vi "DataProcessingDraft.vi"() -> ()   [LabVIEW 2011]
doc: "Processes data from status data logs. Runs through it and finds each time we wrote to the log, and uses the number of times we wrote as the time (time stamps are acting funny). Then allows us to look at various pieces of data and zoom in and out as necessary.\n\n-By Elizabeth Mahon"
uses:
  2-Think/2 Typedefs/logger data.ctl
  2-Think/2 Typedefs/Which Boat.ctl
  2-Think/2 Typedefs/UTM Location.ctl
  2-Think/2 Typedefs/heading.ctl
  2-Think/2 Typedefs/rate of turn.ctl
  2-Think/2 Typedefs/robot velocity.ctl
  2-Think/2 Typedefs/pitch and roll.ctl
  2-Think/2 Typedefs/generalized sensor status.ctl
  2-Think/2 Typedefs/indicator LED.ctl
  2-Think/2 Typedefs/apparent wind direction.ctl
  2-Think/2 Typedefs/apparent wind speed.ctl
  2-Think/2 Typedefs/absolute wind direction.ctl
  2-Think/2 Typedefs/absolute wind speed.ctl
  0x2-OCU-Think Comm/0x2 Typedefs/Current Waypoint.ctl
  2-Think/2 Typedefs/UTM Circle.ctl
  2-Think/2 Typedefs/rudder angle.ctl
  2-Think/2 Typedefs/sail setpt.ctl
  0x2-OCU-Think Comm/0x2 Typedefs/manual override.ctl
  2-Think/2 Typedefs/setpoints to boat.ctl
panel:
  in  "Max time":dbl
  in  "Min time":dbl
  in  "Stop Viewing Data":bool
  in  "Choose graph to display":T1(tab)
  in  "Min Frequency":dbl
  in  "Max Frequency":dbl
  out "Code Speed":cluster{i32[], dbl[]}[](graph)
  out "Location":cluster{dbl[], dbl[]}(graph)
  out "Battery Voltage":cluster{i32[], dbl[]}(graph)
  in  "Min Velocity":dbl
  in  "Max Velocity":dbl
  out "Velocity":cluster{i32[], dbl[]}[](graph)
  in  "Min Angle":dbl
  in  "Max Angle":dbl
  out "Headings":cluster{i32[], dbl[]}[](graph)
  out "Rudder":cluster{i32[], dbl[]}(graph)
  out "Sail":cluster{i32[], dbl[]}(graph)
  in  "Data Log":T2 {"Current Waypoint Coords"."North" format="%#_10f"; "Current Waypoint Coords"."East" format="%#_8f"; "Robot Pitch/Roll"."Roll" format="%05.1f"; "Robot Pitch/Roll"."Pitch" format="%05.1f"; "Robot\nRate of Turn" format="%05.1f"; "Robot\nHeading" format="%05.1f"; "Robot UTM Location"."North" format="%#_10f"; "Robot UTM Location"."East" format="%#_8f"}
  # "Act and network frequency are always 0.\nAs far as I can tell, network frequency is never set, so of course it's 0.\nAct, while set, is in a sequence structure where the first frame has a while loop that only ends if we e-stop, so it'll never get set."
  # "Where Am I?"
  # "Path Planning"
  # "From Planning Functions"
  # "(this is not a cluster because subitems\nare generated in parallel code)"
  # "How Am I?"
  # "What's Around Me?"
  # "As Measured"
  # "As Measured"
  # "Loop Rates"
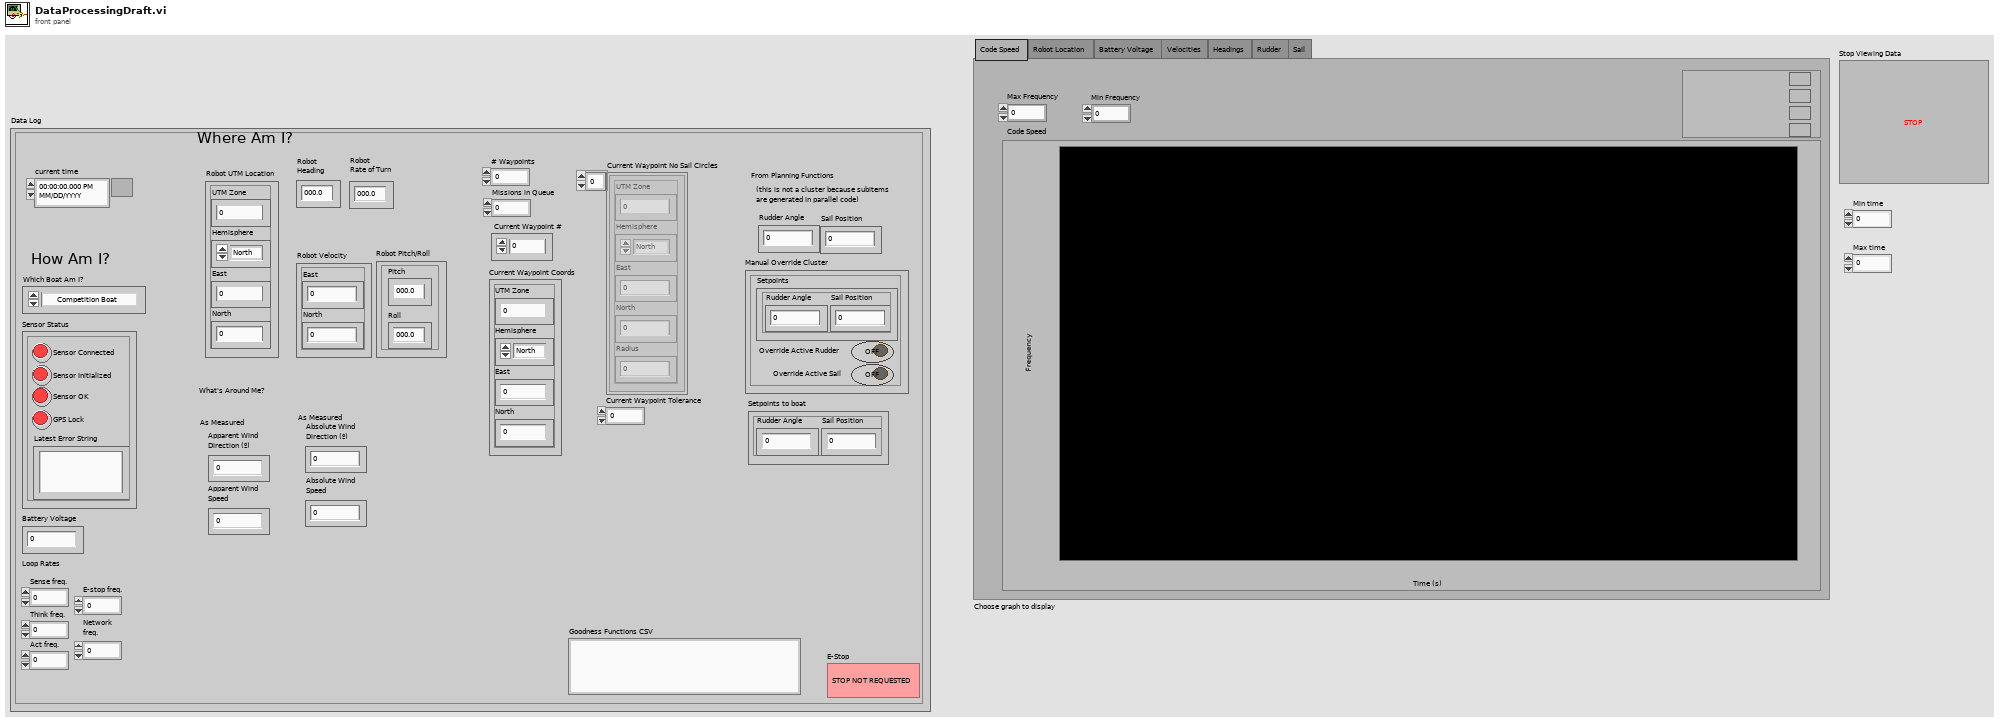
[diagram p1: front panel]
types:
  T1 = enum32{"Code Speed", "Robot Location", "Battery Voltage", "Velocities", "Headings", "Rudder", "Sail"}
  T2 = typedef "logger data.ctl" = cluster{"current time":timestamp, "Which Boat Am I?":T3, "Robot UTM Location":T4, "Robot\nHeading ":T5, "Robot\nRate of Turn":T6, "Robot Velocity":T7, "Robot Pitch/Roll":T8, "Sensor Status":T9, "Battery Voltage":dbl, "Sense freq.":dbl, "Think freq.":dbl, "Act freq.":dbl, "E-stop freq.":dbl, "Network \nfreq.":dbl, "Apparent Wind\nDirection (º)":T11, "Apparent Wind\nSpeed":T12, "Absolute Wind\nDirection (º)":T13, "Absolute Wind\nSpeed":T14, "Missions in Queue":i32, "# Waypoints":i32, " Current Waypoint #":T15, "Current Waypoint Coords":T4, "Current Waypoint Tolerance":dbl, "Current Waypoint No Sail Circles":T16[], "Rudder Angle":T17, "Sail Position":T18, "Manual Override Cluster":T19, "Setpoints to boat":T20, "E-Stop":bool, "Goodness Functions CSV":string}
  T3 = typedef "Which Boat.ctl" = enum16{"Competition Boat", "Small RC", "Simulation"}
  T4 = typedef "UTM Location.ctl" = cluster{"UTM Zone":dbl, "Hemisphere":enum16{"North", "South"}, "East":dbl, "North":dbl}
  T5 = typedef "heading.ctl" = dbl
  T6 = typedef "rate of turn.ctl" = dbl
  T7 = typedef "robot velocity.ctl" = cluster{"East":dbl, "North":dbl}
  T8 = typedef "pitch and roll.ctl" = cluster{"Pitch":dbl, "Roll":dbl}
  T9 = typedef "generalized sensor status.ctl" = cluster{"Sensor Connected":T10, "Sensor Initialized":T10, "Sensor OK":T10, "Latest Error String":string, "GPS Lock":T10}
  T10 = typedef "indicator LED.ctl" = bool
  T11 = typedef "apparent wind direction.ctl" = dbl
  T12 = typedef "apparent wind speed.ctl" = dbl
  T13 = typedef "absolute wind direction.ctl" = dbl
  T14 = typedef "absolute wind speed.ctl" = dbl
  T15 = typedef "Current Waypoint.ctl" = i32
  T16 = typedef "UTM Circle.ctl" = cluster{"UTM Zone":dbl, "Hemisphere":enum16{"North", "South"}, "East":dbl, "North":dbl, "Radius":dbl}
  T17 = typedef "rudder angle.ctl" = dbl
  T18 = typedef "sail setpt.ctl" = dbl
  T19 = typedef "manual override.ctl" = cluster{"Override Active Rudder":bool, "Setpoints":T20, "Override Active Sail":bool}
  T20 = typedef "setpoints to boat.ctl" = cluster{"Sail Position":T18, "Rudder Angle":T17}
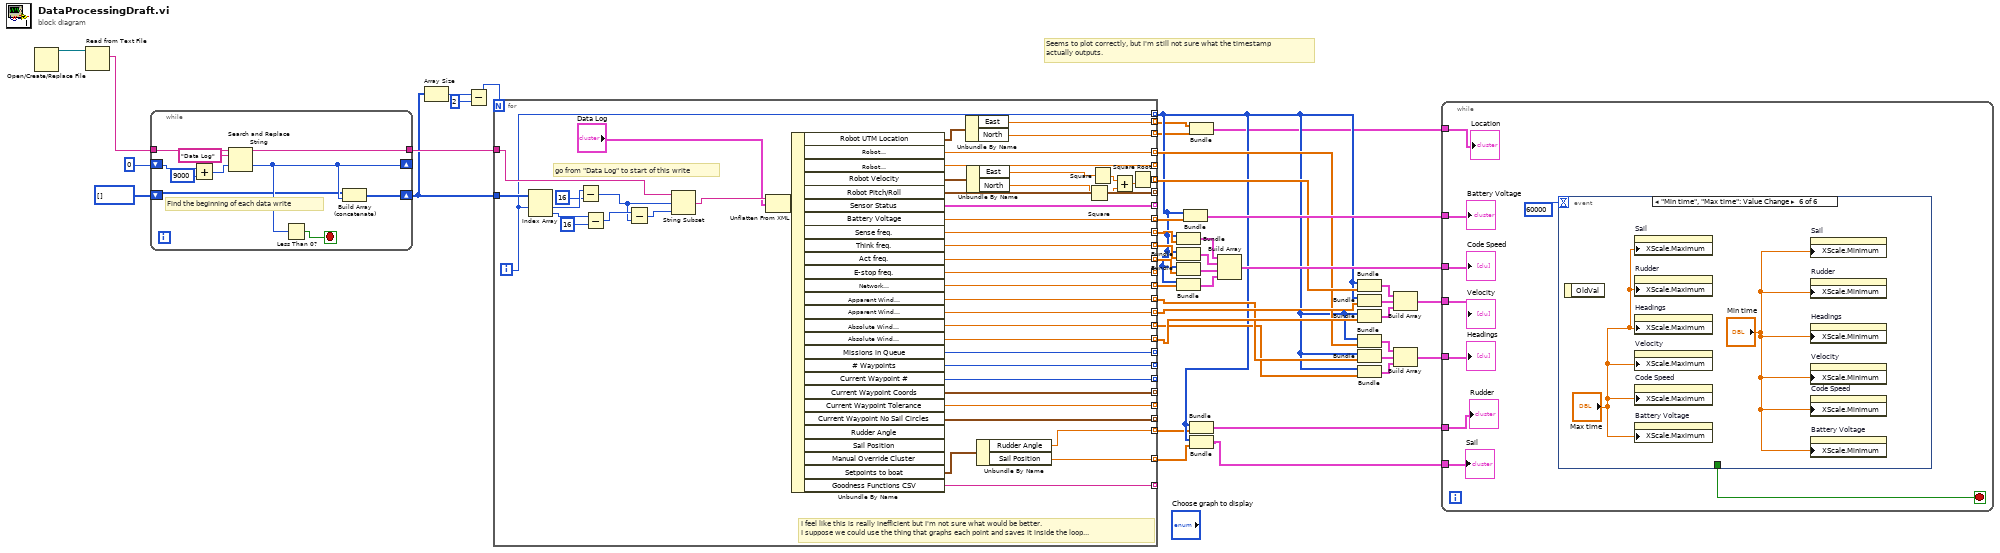
[diagram p0: block diagram]
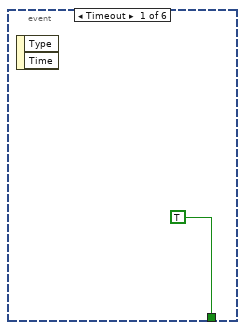
[diagram p2: hidden frame]
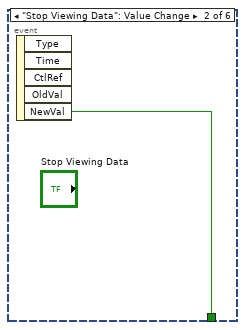
[diagram p3: hidden frame]
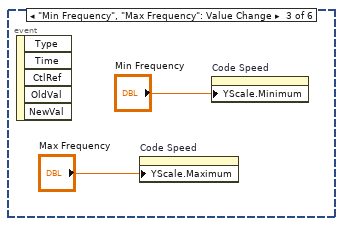
[diagram p4: hidden frame]
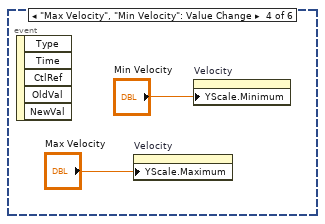
[diagram p5: hidden frame]
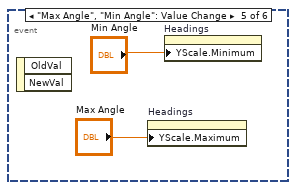
[diagram p6: hidden frame]
diagram:
  # "Seems to plot correctly, but I'm still not sure what the timestamp\nactually outputs."
  n1 = Open/Create/Replace File() -> (refnum out=w42:refnum<file>)  [unwired: 6 in, 2 out]
  n2 = Read from Text File(file (use dialog)=w42) -> (text=w41:string)  [unwired: 3 in, 3 out]
  n3 = while {
    tunnel: w41 -> [w51]
    shift-right: [w46] -> _
    shift-left: 0 ("offset past replacement") -> [w50]
    shift-right: [w45] -> w37
    shift-left: i32[] [] -> [w44]
    tunnel: [w43] -> w38
    stop <- w47 stop-if-true
    # "Find the beginning of each data write"
    n4 = Add(x=w50, y=9000) -> (x+y=w48:i32)
    n5 = Search and Replace String(input string=w51, search string="Data Log", offset=w48) -> (result string=w43:string, offset past replacement=w46:i32)  [unwired: 5 in, 2 out]
    n6 = Less Than 0?(x=w46) -> (x < 0?=w47:bool)
    n7 = Build Array (concatenate)(w44, w46) -> (w45:i32[])
  }
  n8 = Array Size(array=w37) -> (size(s)=w36:i32)
  n9 = Subtract(x=w36, y=2) -> (x-y=w35:i32)
  n10 = for {
    N: w35 -> [_]
    tunnel: w37 -> [w91]
    tunnel: w38 -> [w94]
    tunnel: [w87] -> w12 mode=indexing
    tunnel: [w86] -> _ mode=indexing
    tunnel: [w85] -> _ mode=indexing
    tunnel: [w84] -> _ mode=indexing
    tunnel: [w83] -> w23 mode=indexing
    tunnel: [w82] -> w21 mode=indexing
    tunnel: [w81] -> w20 mode=indexing
    tunnel: [w80] -> w19 mode=indexing
    tunnel: [w79] -> _ mode=indexing
    tunnel: [w78] -> w18 mode=indexing
    tunnel: [w77] -> w11 mode=indexing
    tunnel: [w76] -> w15 mode=indexing
    tunnel: [w75] -> w10 mode=indexing
    tunnel: [w74] -> w14 mode=indexing
    tunnel: [w73] -> _ mode=indexing
    tunnel: [w72] -> _ mode=indexing
    tunnel: [w71] -> _ mode=indexing
    tunnel: [w70] -> _ mode=indexing
    tunnel: [w69] -> _ mode=indexing
    tunnel: [w68] -> _ mode=indexing
    tunnel: [w67] -> _ mode=indexing
    tunnel: [w66] -> w9 mode=indexing
    tunnel: [w59] -> w16 mode=indexing
    tunnel: [w57] -> w7 mode=indexing
    tunnel: [w56] -> w6 mode=indexing
    tunnel: [w54] -> w3 mode=indexing
    tunnel: [w53] -> w2 mode=indexing
    i -> [w66]
    # "I feel like this is really inefficient but I'm not sure what would be better.\nI suppose we could use the thing that graphs each point and saves it inside the loop..."
    # "go from \"Data Log\" to start of this write"
    n11 = Index Array(array=w91, index #1=w66) -> (element #1=w99:i32, element #2=w97:i32)  [unwired: 1 in]
    n12 = Subtract(x=w99, y=16) -> (x-y=w92:i32)
    n13 = Subtract(x=w97, y=16) -> (x-y=w95:i32)
    n14 = Subtract(x=w95, y=w92) -> (x-y=w93:i32)
    n15 = String Subset(string=w94, offset (0)=w92, length (rest)=w93) -> (substring=w90:string)
    n16 = Unflatten From XML(xml string=w90, type="Data Log") -> (value=w88:T2)  [unwired: 1 in, 1 out]
    n17 = Unbundle By Name(w88) -> ("Robot UTM Location"=w55:T4, "Robot\nHeading"=w87:T5, "Robot\nRate of Turn"=w86:T6, "Robot Velocity"=w65:T7, "Robot Pitch/Roll"=w85:T8, "Sensor Status"=w84:T9, "Battery Voltage"=w83:dbl, "Sense freq."=w82:dbl, "Think freq."=w81:dbl, "Act freq."=w80:dbl, "E-stop freq."=w79:dbl, "Network \nfreq."=w78:dbl, "Apparent Wind\nDirection (º)"=w77:T11, "Apparent Wind\nSpeed"=w76:T12, "Absolute Wind\nDirection (º)"=w75:T13, "Absolute Wind\nSpeed"=w74:T14, "Missions in Queue"=w73:i32, "# Waypoints"=w72:i32, "Current Waypoint #"=w71:T15, "Current Waypoint Coords"=w70:T4, "Current Waypoint Tolerance"=w69:dbl, "Current Waypoint No Sail Circles"=w68:T16[], "Setpoints to boat"=w58:T20, "Goodness Functions CSV"=w67:string)  [unwired: 3 out]
    n18 = Unbundle By Name(w55) -> ("East"=w54:dbl, "North"=w53:dbl)
    n19 = Unbundle By Name(w65) -> ("East"=w64:dbl, "North"=w63:dbl)
    n20 = Unbundle By Name(w58) -> ("Rudder Angle"=w57:T17, "Sail Position"=w56:T18)
    n21 = Square(x=w63) -> (x^2=w60:dbl)
    n22 = Square(x=w64) -> (x^2=w61:dbl)
    n23 = Add(x=w61, y=w60) -> (x+y=w62:dbl)
    n24 = Square Root(x=w62) -> (sqrt(x)=w59:dbl)
  }
  n25 = Bundle(w9, w21) -> (w25:cluster{i32[], dbl[]})  [unwired: 1 in]
  n26 = Bundle(w9, w20) -> (w24:cluster{i32[], dbl[]})  [unwired: 1 in]
  n27 = Bundle(w9, w19) -> (w27:cluster{i32[], dbl[]})  [unwired: 1 in]
  n28 = Bundle(w9, w18) -> (w26:cluster{i32[], dbl[]})  [unwired: 1 in]
  n29 = Bundle(w9, w23) -> (w22:cluster{i32[], dbl[]})  [unwired: 1 in]
  n30 = Bundle(w3, w2) -> (w1:cluster{dbl[], dbl[]})  [unwired: 1 in]
  n31 = Bundle(w9, w7) -> (w5:cluster{i32[], T17[]})  [unwired: 1 in]
  n32 = Bundle(w9, w6) -> (w4:cluster{i32[], T18[]})  [unwired: 1 in]
  n33 = Build Array(w25, w24, w27, w26) -> (w17:cluster{i32[], dbl[]}[])
  n34 = Bundle(w9, w16) -> (w31:cluster{i32[], dbl[]})  [unwired: 1 in]
  n35 = Bundle(w9, w15) -> (w32:cluster{i32[], T12[]})  [unwired: 1 in]
  n36 = Bundle(w9, w14) -> (w33:cluster{i32[], T14[]})  [unwired: 1 in]
  n37 = Bundle(w9, w12) -> (w28:cluster{i32[], T5[]})  [unwired: 1 in]
  n38 = Bundle(w9, w11) -> (w29:cluster{i32[], T11[]})  [unwired: 1 in]
  n39 = Bundle(w9, w10) -> (w30:cluster{i32[], T13[]})  [unwired: 1 in]
  n40 = Build Array(w31, w32, w33) -> (w13:cluster{i32[], T14[]}[])
  n41 = Build Array(w28, w29, w30) -> (w8:cluster{i32[], T13[]}[])
  n42 = while {
    tunnel: w22 -> [w108]
    tunnel: w17 -> [w107]
    tunnel: w13 -> [w106]
    tunnel: w8 -> [w105]
    tunnel: w5 -> [w102]
    tunnel: w4 -> [w101]
    tunnel: w1 -> [w100]
    stop <- w103 stop-if-true
    n43 = event shown="[5] \"Min time\", \"Max time\": Value Change" {
      selector: _ -> [_ _ _ _ _ _]
      dyn-events: _ -> [_ _ _ _ _ _]
      timeout: 60000 -> [_ _ _ _ _ _]
      tunnel: [TRUE w110 _ _ _ _] -> w103
      event Timeout {
        n44 = event-data() -> ()  [unwired: 1 in, 2 out]
      }
      event "Stop Viewing Data": Value Change {
        n45 = event-data() -> ("NewVal"=w110:bool)  [unwired: 1 in, 4 out]
      }
      event "Min Frequency", "Max Frequency": Value Change {
        n46 = event-data() -> ()  [unwired: 1 in, 5 out]
        n47 = property on="Code Speed" class="XYGraph (strict)"("YScale.Maximum"="Max Frequency") -> ()  [unwired: 2 in, 2 out]
        n48 = property on="Code Speed" class="XYGraph (strict)"("YScale.Minimum"="Min Frequency") -> ()  [unwired: 2 in, 2 out]
      }
      event "Max Velocity", "Min Velocity": Value Change {
        n49 = event-data() -> ()  [unwired: 1 in, 5 out]
        n50 = property on="Velocity" class="XYGraph (strict)"("YScale.Maximum"="Max Velocity") -> ()  [unwired: 2 in, 2 out]
        n51 = property on="Velocity" class="XYGraph (strict)"("YScale.Minimum"="Min Velocity") -> ()  [unwired: 2 in, 2 out]
      }
      event "Max Angle", "Min Angle": Value Change {
        n52 = event-data() -> ()  [unwired: 1 in, 2 out]
        n53 = property on="Headings" class="XYGraph (strict)"("YScale.Maximum"="Max Angle") -> ()  [unwired: 2 in, 2 out]
        n54 = property on="Headings" class="XYGraph (strict)"("YScale.Minimum"="Min Angle") -> ()  [unwired: 2 in, 2 out]
      }
      event "Min time", "Max time": Value Change {
        n55 = event-data() -> ()  [unwired: 1 in, 1 out]
        n56 = property on="Sail" class="XYGraph (strict)"("XScale.Maximum"="Max time") -> ()  [unwired: 2 in, 2 out]
        n57 = property on="Rudder" class="XYGraph (strict)"("XScale.Maximum"="Max time") -> ()  [unwired: 2 in, 2 out]
        n58 = property on="Headings" class="XYGraph (strict)"("XScale.Maximum"="Max time") -> ()  [unwired: 2 in, 2 out]
        n59 = property on="Velocity" class="XYGraph (strict)"("XScale.Maximum"="Max time") -> ()  [unwired: 2 in, 2 out]
        n60 = property on="Code Speed" class="XYGraph (strict)"("XScale.Maximum"="Max time") -> ()  [unwired: 2 in, 2 out]
        n61 = property on="Battery Voltage" class="XYGraph (strict)"("XScale.Maximum"="Max time") -> ()  [unwired: 2 in, 2 out]
        n62 = property on="Sail" class="XYGraph (strict)"("XScale.Minimum"="Min time") -> ()  [unwired: 2 in, 2 out]
        n63 = property on="Rudder" class="XYGraph (strict)"("XScale.Minimum"="Min time") -> ()  [unwired: 2 in, 2 out]
        n64 = property on="Headings" class="XYGraph (strict)"("XScale.Minimum"="Min time") -> ()  [unwired: 2 in, 2 out]
        n65 = property on="Velocity" class="XYGraph (strict)"("XScale.Minimum"="Min time") -> ()  [unwired: 2 in, 2 out]
        n66 = property on="Code Speed" class="XYGraph (strict)"("XScale.Minimum"="Min time") -> ()  [unwired: 2 in, 2 out]
        n67 = property on="Battery Voltage" class="XYGraph (strict)"("XScale.Minimum"="Min time") -> ()  [unwired: 2 in, 2 out]
      }
    }
    "Velocity" <- w106
    "Rudder" <- w102
    "Headings" <- w105
    "Code Speed" <- w107
    "Battery Voltage" <- w108
    "Sail" <- w101
    "Location" <- w100
  }
